vi "Find Message Text QD.vi"(7 "Event Selector Name":string, 8 "error in (no error)":errorcluster, 11 "EventStructure in":refnum<vi>) -> (0 "error out":errorcluster, 5 "Message Text":string)   [LabVIEW 2017]
doc: "Returns the Message text pass from the EHL to the MHL for the event handle by the Event Selectore Name event case."
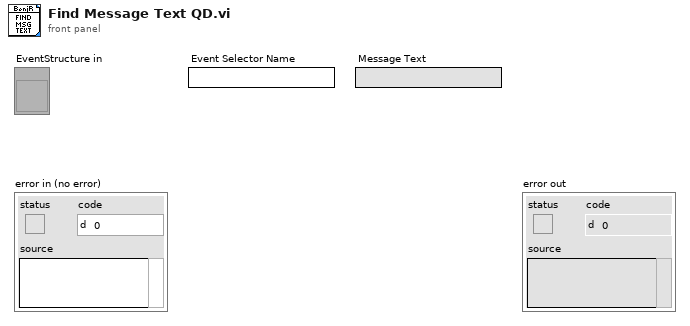
[diagram p1: front panel]
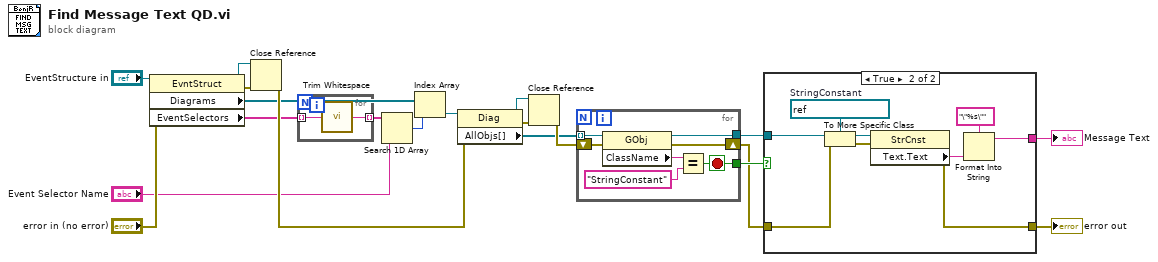
[diagram p0: block diagram]
diagram:
  n1 = property class="EvntStruct"(reference="EventStructure in", error in="error in (no error)") -> (reference out=w14:refnum<vi>, error out=w15:errorcluster, "Diagrams"=w12:refnum<vi>[], "EventSelectors"=w5:string[])
  n2 = Close Reference(reference=w14, error in (no error)=w15) -> (error out=w16:errorcluster)
  n3 = for {
    tunnel: w5 -> [w22] mode=indexing
    tunnel: [w21] -> w6 mode=indexing
    n4 = call <vilib>:"Trim Whitespace.vi"("string"=w22) -> ("trimmed string"=w21:string)  [unwired: 1 in]
  }
  n5 = Search 1D Array(1D array=w6, element="Event Selector Name") -> (index of element=w2:i32)  [unwired: 1 in]
  n6 = Index Array(array=w12, index=w2) -> (element=w3:refnum<vi>)
  n7 = property class="Diag"(reference=w3, error in=w16) -> (reference out=w17:refnum<vi>, error out=w18:errorcluster, "AllObjs[]"=w4:refnum<vi>[])
  n8 = Close Reference(reference=w17, error in (no error)=w18) -> (error out=w19:errorcluster)
  n9 = for {
    tunnel: w4 -> [w29] mode=indexing
    tunnel: [w26] -> w7
    shift-right: [w24] -> w13
    shift-left: w19 -> [w25]
    tunnel: [w23] -> w20
    stop <- w23 stop-if-true
    n10 = property class="GObj"(reference=w29, error in=w25) -> (reference out=w26:refnum<vi>, error out=w24:errorcluster, "ClassName"=w28:string)
    n11 = Equal?(x=w28, y="StringConstant" ("Class Name")) -> (x = y?=w23:bool)
  }
  n12 = case shown="True" w20 {
    tunnel: w7 -> [_ w39]
    tunnel: [_ w34] -> w8
    tunnel: [w30 w33] -> w9
    tunnel: w13 -> [w30 w32]
    frame False {
    }
    frame True {
      w38 = refnum<vi> refnum  # StringConstant
      n13 = To More Specific Class(target class=w38, reference=w39, error in=w32) -> (specific class reference=w37:refnum<vi>, error out=w31:errorcluster)
      n14 = property class="StrCnst"(reference=w37, error in=w31) -> (error out=w33:errorcluster, "Text.Text"=w36:string)  [unwired: 1 out]
      n15 = Format Into String(format string="\"%s\"", w36) -> (resulting string=w34:string)  [unwired: 2 in, 1 out]
    }
  }
  "error out" <- w9
  "Message Text" <- w8
